vi "Yaw_Arb.vi"(0 "P1_Value":dbl, 1 "P1_Enable":bool, 2 "P3_Enable":bool, 5 "P2_Value":dbl, 7 "P3_Value":dbl, 9 "P4_Value":dbl, 12 "P2_Enable":bool, 13 "P4_Enable":bool) -> (4 "P Out":dbl, 6 "Any True?":bool)   [LabVIEW 2015]
panel:
  # "P1 is highest priority\np5 is lowest"
  # "Josh Merkle 2/8/16"
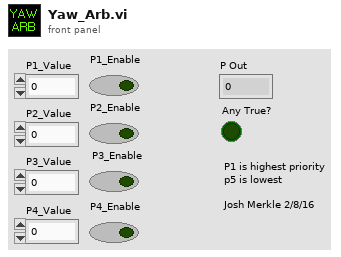
[diagram p1: front panel]
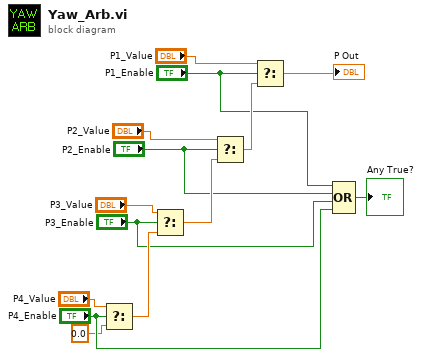
[diagram p0: block diagram]
diagram:
  n1 = Select(t="P4_Value", s="P4_Enable", f=0.0) -> (s? t:f=w14:dbl)
  n2 = Select(t="P3_Value", s="P3_Enable", f=w14) -> (s? t:f=w13:dbl)
  n3 = Select(t="P2_Value", s="P2_Enable", f=w13) -> (s? t:f=w12:dbl)
  n4 = Select(t="P1_Value", s="P1_Enable", f=w12) -> (s? t:f=→"P Out":dbl)
  n5 = Compound Arithmetic op=OR("P1_Enable", "P2_Enable", "P3_Enable", "P4_Enable") -> (→"Any True?":bool)
